vi "BodeMagnitudePlot.vi"   [LabVIEW 2014]
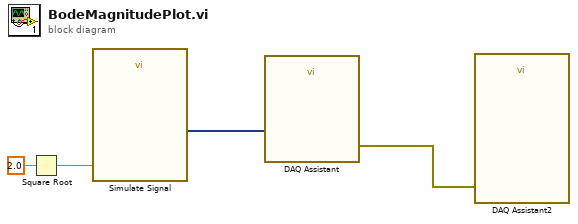
[diagram p0: block diagram]
diagram:
  n1 = Square Root(x=2.0 ("Amplitude")) -> (sqrt(x)=w1:dbl)
  n2 = call "Simulate Signal"("Amplitude"=w1) -> ("Sine"=w4:dynamicdata)  [unwired: 13 in, 1 out]
  n3 = call "DAQ Assistant"("data"=w4) -> ("error out"=w3:errorcluster)  [unwired: 17 in, 1 out]
  n4 = call "DAQ Assistant2"("error in"=w3) -> ()  [unwired: 16 in, 3 out]
